vi "sendFloat32.vi"() -> ()   [LabVIEW 2018, in "LV-0mq-Julia_roundtrip-lib.lvlib" / "LV2Julia_core.lvlib"]
uses:
  LV2Julia_core.lvlib
  Commands.ctl
  example server response cluster.ctl
  commands LV2Jl.ctl
  cb7a600e-1a3f-45a0-9149-1773accb9ab7.vi
  Server or client state.ctl
  5d385633-7562-4640-8300-e9530f023818.vi
  9ad41121-06aa-4420-b411-b77d699816f6.vi
  1dfdb4f7-ca7c-4f7f-81a6-5262bc9fa906.vi
  Julia functions enum.ctl
  d2cb43a9-9305-42fb-ad58-bce983510195.vi
  <vilib>/addons/zeromq/zmq_socket.lvclass
  example args cluster.ctl
panel:
  in  "factor":sgl=1.25 format="%#_13g"
  out "appended array":sgl[][](array[numeric])
  in  "complex add":sgl
  in  "stop LV only":bool
  out "JSON args":string
  out "LV Client state out":T1
  out "Jl Server state out":T1
  out "size(s)":i32
  out "unsigned byte array":u8[](array[numeric])
  out "short err code":u8
  out "flattened array out":sgl[](array[numeric])
  out "parsed response 2":cluster{"nums":dbl[]}
  in  "base":sgl=1.2000002 format="%#_13g"
  in  "go once":bool
  out "JSON out":string
  out "parsed response":T2 {"bin_lng" format="%.0e"}
  in  "arr size":u32=1 min=1
  out "final error":errorcluster
  out "current error":errorcluster
  out "status":string
  in  "stop":bool
  in  "Arguments":T3={"arg1"=1, "arg2"=3.14}
  in  "fun2call":T4
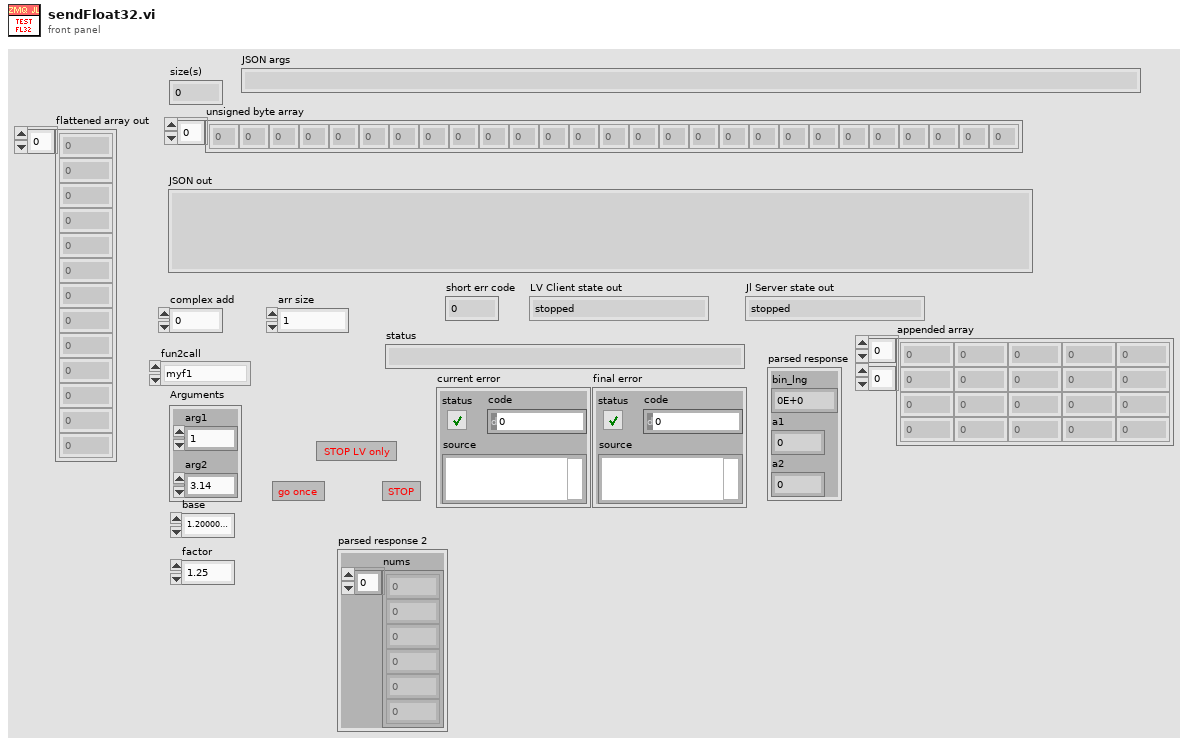
[diagram p1: front panel]
types:
  T1 = typedef "LV-0mq-Julia_roundtrip-lib.lvlib/Server or client state.ctl" = enum16{"stopped", "running", "unknown"}
  T2 = typedef "LV-0mq-Julia_roundtrip-lib.lvlib/example server response cluster.ctl" = cluster{"bin_lng":i32, "a1":i32, "a2":dbl}
  T3 = typedef "LV-0mq-Julia_roundtrip-lib.lvlib/example args cluster.ctl" = cluster{"arg1":i32, "arg2":dbl}
  T4 = typedef "Julia functions enum.ctl" = enum16{"myf1", "myf2", "myf3", "test_bin2nums", "test_rgbimg", "numarr_loopback", "numarrs_lpbk", "Not_a_Fun"}
  T5 = typedef "LV-0mq-Julia_roundtrip-lib.lvlib/Commands.ctl" = enum16{"Start Jl-server & Init LV-client", "Send request & Get response ", "Stop Jl-server & Cleanup LV-client", "Cleanup LV-client", "Start Jl-server", "Stop Jl-server", "Init LV-Client", "Cleanup LV-Client", "(not allowed)", "Set LV Client state", "Set Jl Server state", "set ZMQ timeout", "read ZMQ timeout", "read-out state"}
  T6 = typedef "LV-0mq-Julia_roundtrip-lib.lvlib/commands LV2Jl.ctl" = u8
  T7 = typedef "LV-0mq-Julia_roundtrip-lib.lvlib/Bindata&description.ctl" = cluster{"bindata_descr":T8[], "bindata":u8[]}
  T8 = typedef "LV-0mq-Julia_roundtrip-lib.lvlib/Bindata description.ctl" = cluster{"nofbytes":i32, "numtype":string, "start":i32, "arrdims":i32[], "kwarg_name":string, "category":string}
  T9 = typedef "LV-0mq-Julia_roundtrip-lib.lvlib/detailed error info.ctl" = cluster{"exception_or_info":string, "trace":T10[]}
  T10 = typedef "LV-0mq-Julia_roundtrip-lib.lvlib/StackFrame.ctl" = cluster{"frame_summary":string, "func":string, "linfo":string, "file":string, "line":i32, "pointer":u64, "from_c":bool, "inlined":bool}
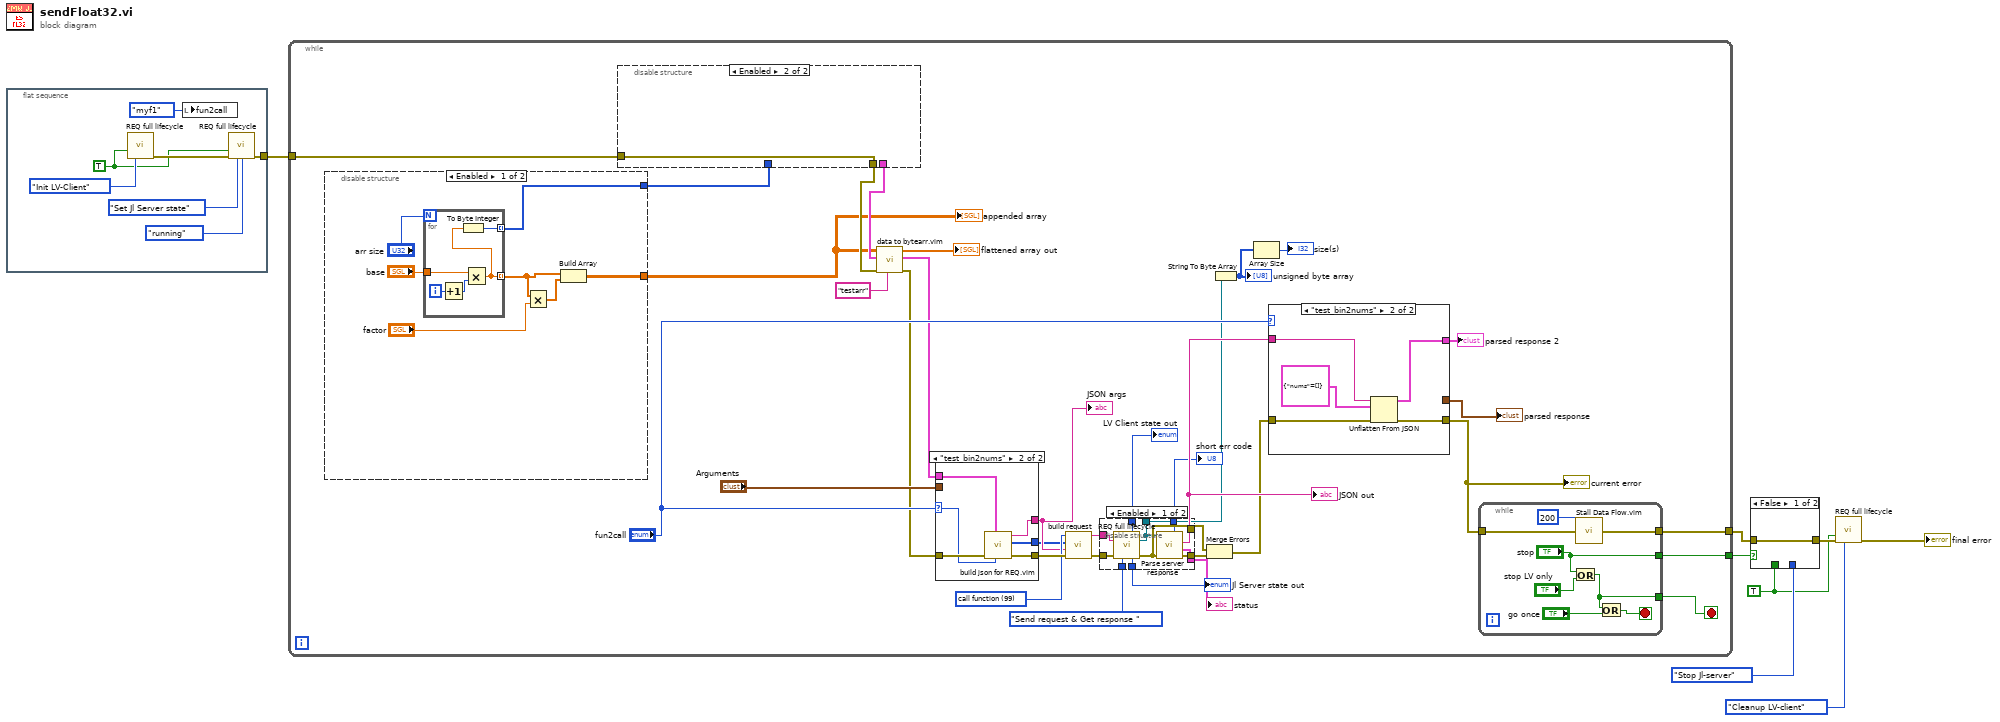
[diagram p0: block diagram]
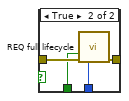
[diagram p2: hidden frame]
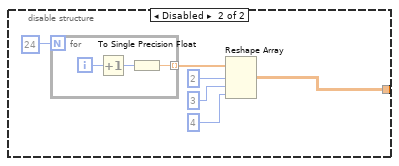
[diagram p3: hidden frame]
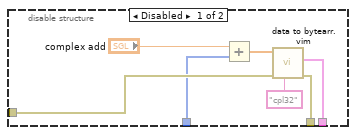
[diagram p4: hidden frame]
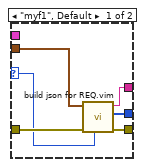
[diagram p6: hidden frame]
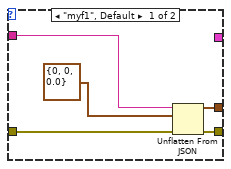
[diagram p7: hidden frame]
diagram:
  w3 = TRUE ("Force command")
  n1 = flat-sequence {
    tunnel: [w13] -> w2
    frame #0 {
      w11 = TRUE ("Force command")
      n2 = call "REQ full lifecycle.vi"("Force command"=w11, "command"=Commands."Init LV-Client") -> ("error out"=w14:errorcluster)  [unwired: 7 in, 6 out]
      n3 = local write "fun2call"(Julia_functions_enum."myf1" ("fun2call")) -> ()
      n4 = call "REQ full lifecycle.vi"("Force command"=w11, "error in"=w14, "command"=Commands."Set Jl Server state", "Jl Server state in"=Server_or_client_state."running") -> ("error out"=w13:errorcluster)  [unwired: 5 in, 6 out]
    }
  }
  n5 = while {
    tunnel: w2 -> [w23]
    tunnel: [w40] -> w8
    tunnel: [w19] -> w1
    stop <- w39 stop-if-true
    w37 = T6 99 items=["call function"=99, "ping"=112, "stop"=115] ("Command")
    n6 = disable-structure shown="Enabled" {
      disable-tunnel: [w56 _] -> w20
      disable-tunnel: [w55 w63] -> w18
      frame Enabled {
        n7 = for {
          N: "arr size" -> [_]
          tunnel: "base" -> [w62]
          tunnel: [w59] -> w54 mode=indexing
          tunnel: [w58] -> w56 mode=indexing
          i -> [w61]
          n8 = Increment(x=w61) -> (x+1=w60:i32)
          n9 = Multiply(x=w62, y=w60) -> (x*y=w59:sgl)
          n10 = To Byte Integer(number=w59) -> (8bit integer=w58:i8)
        }
        n11 = Multiply(x=w54, y="factor") -> (x*y=w53:sgl[])
        n12 = Build Array(w54, w53) -> (w55:sgl[][])
      }
      frame Disabled {
        n13 = for {
          N: 24 -> [_]
          tunnel: [w69] -> w67 mode=indexing
          i -> [w71]
          n14 = Increment(x=w71) -> (x+1=w70:i32)
          n15 = To Single Precision Float(number=w70) -> (single precision float=w69:sgl)
        }
        n16 = Reshape Array(w67, 2 ("dimension size"), 3 ("dimension size"), 4 ("dimension size")) -> (w63:sgl[][][])
      }
    }
    "appended array" <- w18
    n17 = disable-structure shown="Enabled" {
      disable-tunnel: w23 -> [w77 w79]
      disable-tunnel: [w76 w79] -> w22
      disable-tunnel: [w75 _] -> w21
      disable-tunnel: w20 -> [w72 _]
      frame Disabled {
        n18 = Add(x="complex add", y=w72) -> (x+y=w73:sgl[])
        n19 = call "data to bytearr.vim"("kwarg_name"="cpl32" ("Tag"), "error in (no error)"=w77, "data in"=w73) -> ("error out"=w76:errorcluster, "Bindata & descr out"=w75:T7)  [unwired: 6 in, 1 out]
      }
      frame Enabled {
      }
    }
    n20 = call "data to bytearr.vim"("kwarg_name"="testarr" ("Tag"), "error in (no error)"=w22, "Bindata & descr in"=w21, "data in"=w18) -> ("error out"=w33:errorcluster, "Bindata & descr out"=w32:T7, "flattened data out"=→"flattened array out":sgl[])  [unwired: 5 in]
    n21 = case shown="\"test_bin2nums\"" "fun2call" {
      selector: "fun2call" -> [w91 w98]
      tunnel: [w95 w101] -> w47
      tunnel: [w94 w100] -> w17
      tunnel: w33 -> [w96 w102]
      tunnel: "Arguments" -> [w93 _]
      tunnel: [w92 w99] -> w16
      tunnel: w32 -> [_ w97]
      frame "myf1", Default {
        n22 = call "build json for REQ.vim"("fun2call"=w91, "error in (no error)"=w96, "Arguments 1"=w93) -> ("error out"=w95:errorcluster, "bindata out"=w92:u8[], "JSON string out"=w94:string)  [unwired: 6 in]
      }
      frame "test_bin2nums" {
        n23 = call "build json for REQ.vim"("fun2call"=w98, "Bindata & descr in"=w97, "error in (no error)"=w102) -> ("error out"=w101:errorcluster, "bindata out"=w99:u8[], "JSON string out"=w100:string)  [unwired: 6 in]
      }
    }
    "JSON args" <- w17
    n24 = call "build request.vi"("error in (no error)"=w47, "JSON data"=w17, "binary data"=w16, "Command"=w37) -> ("error out"=w45:errorcluster, "REQ string"=w46:string)  [unwired: 6 in]
    n25 = disable-structure shown="Enabled" {
      disable-tunnel: [w90 _] -> w50
      disable-tunnel: [w89 _] -> w49
      disable-tunnel: w46 -> [w88 _]
      disable-tunnel: w45 -> [w87 _]
      disable-tunnel: [w86 _] -> w44
      disable-tunnel: [w85 _] -> w43
      disable-tunnel: Commands."Send request & Get response " ("command") -> [w84 _]
      disable-tunnel: [w83 _] -> w29
      disable-tunnel: [w82 _] -> w28
      disable-tunnel: [w81 _] -> w25
      disable-tunnel: [w80 _] -> w24
      frame Enabled {
        n26 = call "REQ full lifecycle.vi"("data to send"=w88, "error in"=w87, "command"=w84) -> ("LV Client state out"=w80:T1, "socket out"=w82:refnum<class "zmq_socket.lvclass">, "Jl Server state out"=w81:T1, "error out"=w85:errorcluster)  [unwired: 6 in, 3 out]
        n27 = call "Parse server response.vi"("error in (no error)"=w85, "server response in"=w82) -> ("error out"=w86:errorcluster, "detailed error info"=w90:T9, "JSON out"=w89:string, "return code"=w83:u8)  [unwired: 2 in, 4 out]
      }
      frame Disabled {
      }
    }
    "status" <- w50
    "JSON out" <- w49
    "short err code" <- w29
    "Jl Server state out" <- w25
    "LV Client state out" <- w24
    n28 = Merge Errors(w43, w44) -> (w48:errorcluster)
    n29 = String To Byte Array(string=w28) -> (unsigned byte array=w27:u8[])
    "unsigned byte array" <- w27
    n30 = Array Size(array=w27) -> (size(s)=→"size(s)":i32)
    n31 = case shown="\"test_bin2nums\"" "fun2call" {
      tunnel: w49 -> [w115 w120]
      tunnel: w48 -> [w114 w119]
      tunnel: [w113 w118] -> w41
      tunnel: [w112 _] -> w38
      tunnel: [_ w116] -> w36
      frame "myf1", Default {
        n32 = Unflatten From JSON(JSON string=w115, type and defaults=T2 {"bin_lng"=0, "a1"=0, "a2"=0.0} ("parsed response"), error in (no error)=w114) -> (value=w112:T2, error out=w113:errorcluster)  [unwired: 4 in]
      }
      frame "test_bin2nums" {
        n33 = Unflatten From JSON(JSON string=w120, type and defaults=cluster{"nums":dbl[]} {"nums"=[]} ("parsed response"), error in (no error)=w119) -> (value=w116:cluster{"nums":dbl[]}, error out=w118:errorcluster)  [unwired: 4 in]
      }
    }
    "current error" <- w41
    "parsed response" <- w38
    "parsed response 2" <- w36
    n34 = while {
      tunnel: w41 -> [w110]
      tunnel: [w109] -> w40
      tunnel: [w105] -> w39
      tunnel: ["stop"] -> w19
      stop <- w106 stop-if-true
      n35 = Or(x="stop", y="stop LV only") -> (x .or. y?=w105:bool)
      n36 = call "Stall Data Flow.vim"("value in"=w110, "milliseconds to wait"=u32 200) -> ("value out"=w109:errorcluster)  [unwired: 1 out]
      n37 = Or(x=w105, y="go once") -> (x .or. y?=w106:bool)
    }
  }
  n38 = case shown="False" w1 {
    tunnel: w8 -> [w121 w125]
    tunnel: Commands."Stop Jl-server" ("command") -> [_ w124]
    tunnel: [w121 w123] -> w6
    tunnel: w3 -> [_ w122]
    frame False {
    }
    frame True {
      n39 = call "REQ full lifecycle.vi"("Force command"=w122, "error in"=w125, "command"=w124) -> ("error out"=w123:errorcluster)  [unwired: 6 in, 6 out]
    }
  }
  n40 = call "REQ full lifecycle.vi"("Force command"=w3, "error in"=w6, "command"=Commands."Cleanup LV-client") -> ("error out"=→"final error":errorcluster)  [unwired: 6 in, 6 out]
